vi "move_channel.vi"(4 "file index":i32=1, 6 "Mount Channel":i32=1, 8 "Desired":dbl, 9 "Device ID":refnum<vi>, 10 "Serial #":refnum<vi>, 11 "DAQ Channel":tag) -> (1 "Relative Position":waveform(dbl)[](graph) caption="Sensor Sampling", 2 "Absolute vs. Desired Position":cluster{dbl, "Position":dbl}(graph) caption="Waveform Chart", 3 "Absolute Position":dbl)   [LabVIEW 2020]
uses:
  <vilib>/Analysis/NI_AALBase.lvlib
  C:/Users/359167/Documents/LabVIEW_ws/Thorlabs.MotionControl.KCube.InertialMotorCLI.dll
  359167/Documents/LabVIEW_ws/Thorlabs.MotionControl.KCube.InertialMotorCLI.dll
  <vilib>/DAQmx/configure/timing.llb/DAQmx Timing (Sample Clock).vi
  <vilib>/DAQmx/create/channels.llb/DAQmx Create Channel (AI-Voltage-Basic).vi
  <vilib>/Utility/file.llb/Read Delimited Spreadsheet (DBL).vi
  <vilib>/Analysis/baseanly.llb/Mean (DBL).vi
  <vilib>/DAQmx/read.llb/DAQmx Read (Analog 1D Wfm NChan NSamp).vi
panel:
  out "s? t:f":string
  out "Absolute":dbl
  out "Relative (deg.)":dbl
  out "Step Size":i32
  out "Error (deg.)":dbl format="%#.3f"
  in  "Path":path=path "C:/Users/359167/Documents/saved_position.csv"
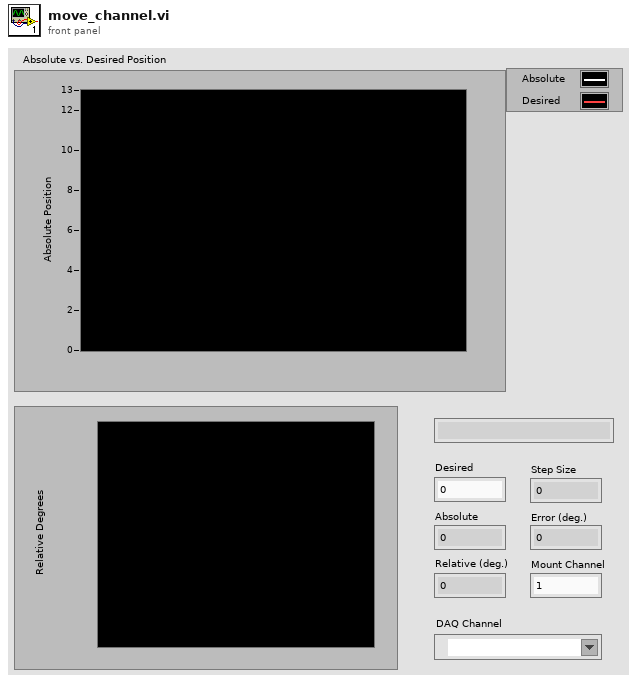
[diagram p1: front panel]
types:
  T1 = cluster{"Absolute Pos.":dbl, "Previous Deg.":dbl}
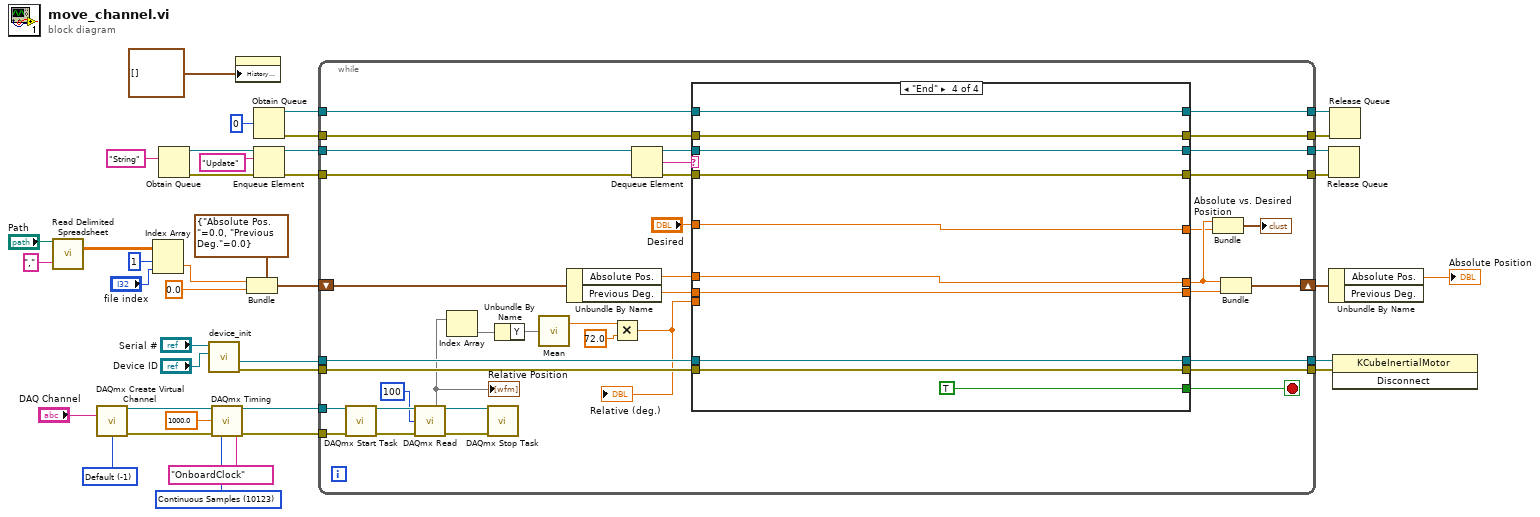
[diagram p0: block diagram]
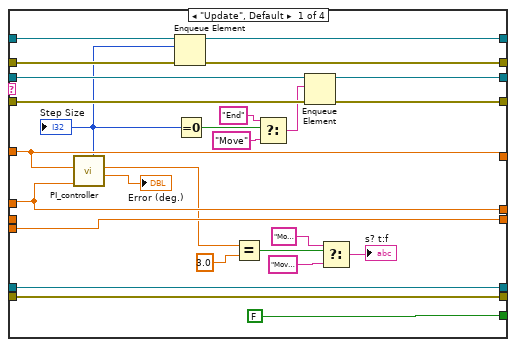
[diagram p2: hidden frame]
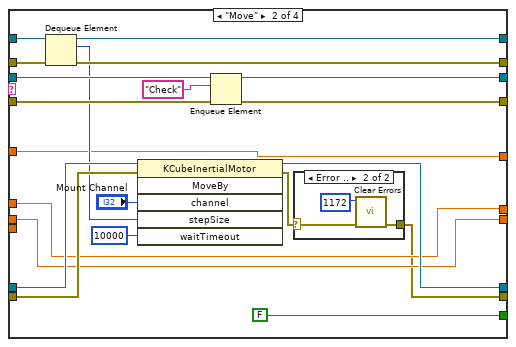
[diagram p3: hidden frame]
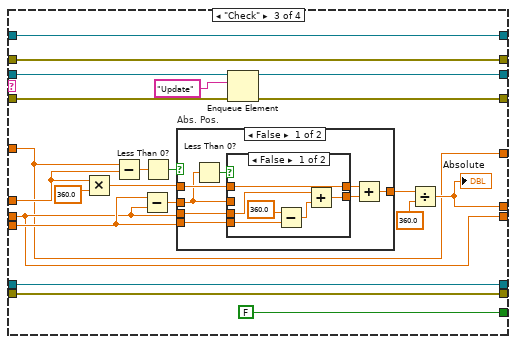
[diagram p5: hidden frame]
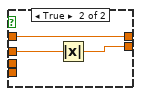
[diagram p6: hidden frame]
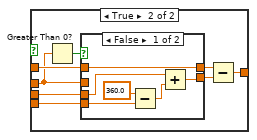
[diagram p7: hidden frame]
diagram:
  w29 = -1 items=["Default"=-1, "RSE"=10083, "NRSE"=10078, "Differential"=10106, "Pseudodifferential"=12529] ("input terminal configuration")
  w30 = 10123 items=["Finite Samples"=10178, "Continuous Samples"=10123, "Hardware Timed Single Point"=12522] ("sample mode")
  n1 = call-poly <vilib>:"Read Delimited Spreadsheet.vi"("file path (dialog if empty)"="Path", "delimiter (\\t)"="," ("delimiter (\\t)")) -> ("all rows"=w33:dbl[][])  [unwired: 8 in, 5 out]
  n2 = call-poly <vilib>:"DAQmx Create Virtual Channel.vi"("input terminal configuration"=w29, "physical channels"="DAQ Channel") -> ("task out"=w25:refnum<k21>, "error out"=w26:errorcluster)  [unwired: 12 in]
  n3 = Index Array(array=w33, index (row)=1, index (col)="file index") -> (element=w18:dbl)
  n4 = Obtain Queue(element data type="String") -> (queue out=w37:refnum<queue>, error out=w36:errorcluster)  [unwired: 4 in, 1 out]
  n5 = call "device_init.vi"("Device ID"="Device ID", "Serial #"="Serial #") -> ("error out"=w6:errorcluster, ".NET Refnum out"=w7:refnum<k24>)  [unwired: 8 in]
  n6 = call-poly <vilib>:"DAQmx Timing.vi"("task/channels in"=w25, "sample mode"=w30, "rate"=1000.0 ("sample rate"), "source"=tag "OnboardClock", "error in"=w26) -> ("task out"=w16:refnum<k21>, "error out"=w15:errorcluster)  [unwired: 9 in]
  n7 = property on="Absolute vs. Desired Position" class="WFChart (strict)"("History Data"=cluster{dbl, "Position":dbl}[] []) -> ()  [unwired: 2 in, 2 out]
  n8 = Bundle(cluster=T1 {"Absolute Pos."=0.0, "Previous Deg."=0.0}, "Absolute Pos."=w18, "Previous Deg."=0.0) -> (w17:T1)
  n9 = Obtain Queue(element data type=0) -> (queue out=w23:refnum<queue>, error out=w22:errorcluster)  [unwired: 4 in, 1 out]
  n10 = Enqueue Element(queue=w37, element="Update", error in (no error)=w36) -> (queue out=w21:refnum<queue>, error out=w20:errorcluster)  [unwired: 1 in, 1 out]
  n11 = while {
    tunnel: w23 -> [w45]
    tunnel: w22 -> [w46]
    tunnel: w20 -> [w59]
    tunnel: [w71] -> w10
    tunnel: [w62] -> w14
    tunnel: [w58] -> w13
    tunnel: [w57] -> w11
    tunnel: w21 -> [w60]
    tunnel: w16 -> [w74]
    tunnel: w15 -> [w73]
    shift-right: [w56] -> w12
    shift-left: w17 -> [w51]
    tunnel: w7 -> [w55]
    tunnel: [w72] -> w5
    tunnel: w6 -> [w54]
    tunnel: [w47] -> w4
    stop <- w76 stop-if-true
    # "Consumer"
    n12 = call <vilib>:"DAQmx Start Task.vi"("task/channels in"=w74, "error in"=w73) -> ("task out"=w67:refnum<k21>, "error out"=w68:errorcluster)  [unwired: 12 in]
    n13 = call-poly <vilib>:"DAQmx Read.vi"("task/channels in"=w67, "number of samples per channel"=100 ("n samples/channel"), "error in"=w68) -> (3:w42, "task out"=w69:refnum<k21>, "error out"=w70:errorcluster)  [unwired: 9 in, 1 out]
    "Relative Position" <- w42
    n14 = Index Array(array=w42) -> (element=w65)  [unwired: 1 in]
    n15 = call <vilib>:"DAQmx Stop Task.vi"("task/channels in"=w69, "error in"=w70) -> ()  [unwired: 12 in, 2 out]
    n16 = Unbundle By Name ("Get Waveform Components")(w65) -> ("Y"=w64)
    n17 = call-poly <vilib>:"Mean.vi"("X"=w64) -> ("mean"=w41:dbl)  [unwired: 1 out]
    n18 = Unbundle By Name(w51) -> ("Absolute Pos."=w48:dbl, "Previous Deg."=w49:dbl)
    n19 = Multiply(x=w41, y=72.0) -> (x*y=w52:dbl)
    "Relative (deg.)" <- w52
    n20 = Dequeue Element(queue=w60, error in (no error)=w59) -> (queue out=w78:refnum<queue>, element=w77:string, error out=w75:errorcluster)  [unwired: 1 in, 1 out]
    n21 = case shown="\"End\"" w77 {
      tunnel: w78 -> [w98 w124 w148 w191]
      tunnel: [w104 w119 w149 w192] -> w71
      tunnel: [FALSE FALSE FALSE TRUE] -> w76
      tunnel: w75 -> [w103 w122 w147 w192]
      tunnel: w45 -> [w102 w110 w146 w193]
      tunnel: w46 -> [w101 w109 w145 w190]
      tunnel: [w100 w108 w146 w193] -> w62
      tunnel: [w99 w107 w145 w190] -> w58
      tunnel: [w90 w125 w134 w187] -> w72
      tunnel: [w91 w112 w135 w188] -> w47
      tunnel: [w94 w121 w150 w191] -> w57
      tunnel: [w88 w114 w140 w189] -> w53
      tunnel: [w89 w113 w131 w185] -> w50
      tunnel: w55 -> [w90 w116 w134 w187]
      tunnel: w54 -> [w91 w115 w135 w188]
      tunnel: "Desired" -> [w87 w105 w130 w186]
      tunnel: w52 -> [w89 _ w133 _]
      tunnel: w48 -> [w88 w114 w132 w189]
      tunnel: w49 -> [_ w113 w131 w185]
      tunnel: [w87 w105 w130 w186] -> w43
      frame "Update", Default {
        n22 = call "PI_controller.vi"("absolute"=w88, "desired"=w87) -> ("degree error"=→"Error (deg.)":dbl, "direction"=w79:dbl, "step size"=w81:i32)  [unwired: 7 in]
        "Step Size" <- w81
        n23 = Enqueue Element(queue=w102, element=w81, error in (no error)=w101) -> (queue out=w100:refnum<queue>, error out=w99:errorcluster)  [unwired: 1 in, 1 out]
        n24 = Equal To 0?(x=w81) -> (x = 0?=w93:bool)
        n25 = Equal?(x=w79, y=3.0) -> (x = y?=w83:bool)
        n26 = Select(t="End", s=w93, f="Move" ("element")) -> (s? t:f=w95:string)
        n27 = Enqueue Element(queue=w98, element=w95, error in (no error)=w103) -> (queue out=w94:refnum<queue>, error out=w104:errorcluster)  [unwired: 1 in, 1 out]
        n28 = Select(t="Moving in reverse direction . . .", s=w83, f="Moving in forward direction . . .") -> (s? t:f=→"s? t:f":string)
      }
      frame "Move" {
        n29 = Dequeue Element(queue=w110, error in (no error)=w109) -> (queue out=w108:refnum<queue>, element=w106:i32, error out=w107:errorcluster)  [unwired: 1 in, 1 out]
        n30 = invoke class="KCubeInertialMotor" method="MoveBy"(reference=w116, error in=w115, "channel"="Mount Channel", "stepSize"=w106, "waitTimeout"=10000) -> (reference out=w125:refnum<k24>, error out=w111:errorcluster)  [unwired: 1 in, 4 out]
        n31 = Enqueue Element(queue=w124, element="Check", error in (no error)=w122) -> (queue out=w121:refnum<queue>, error out=w119:errorcluster)  [unwired: 1 in, 1 out]
        n32 = case shown="Error .." w111 {
          selector: w111 -> [w126 w128]
          tunnel: [w126 w127] -> w112
          frame No Error {
          }
          frame Error {
            n33 = call <vilib>:"Clear Errors.vi"("error in (no error)"=w128, "specific error code to clear (0: all)"=1172) -> ("error out"=w127:errorcluster)  [unwired: 4 in, 1 out]
          }
        }
      }
      frame "Check" {
        n34 = Multiply(x=w132, y=360.0) -> (x*y=w136:dbl)
        n35 = Subtract(x=w130, y=w132) -> (x-y=w139:dbl)
        n36 = Subtract(x=w133, y=w131) -> (x-y=w138:dbl)
        n37 = Less Than 0?(x=w139) -> (x < 0?=w143:bool)
        n38 = case "Abs. Pos." shown="False" w143 {
          tunnel: w136 -> [w156 w176]
          tunnel: w131 -> [w158 w174]
          tunnel: [w157 w172] -> w142
          tunnel: w133 -> [w153 w170]
          tunnel: w138 -> [w152 w169]
          frame False {
            n39 = Less Than 0?(x=w152) -> (x < 0?=w159:bool)
            n40 = case shown="False" w159 {
              tunnel: w156 -> [w165 w168]
              tunnel: [w160 w166] -> w154
              tunnel: w158 -> [w161 _]
              tunnel: w153 -> [w163 _]
              tunnel: [w165 w168] -> w155
              tunnel: w152 -> [_ w167]
              frame False {
                n41 = Subtract(x=360.0 ("y"), y=w163) -> (x-y=w162:dbl)
                n42 = Add(x=w161, y=w162) -> (x+y=w160:dbl)
              }
              frame True {
                n43 = Absolute Value(x=w167) -> (abs(x)=w166:dbl)
              }
            }
            n44 = Add(x=w155, y=w154) -> (x+y=w157:dbl)
          }
          frame True {
            n45 = Greater Than 0?(x=w169) -> (x > 0?=w175:bool)
            n46 = case shown="False" w175 {
              tunnel: w176 -> [w179 w184]
              tunnel: w169 -> [_ w183]
              tunnel: w174 -> [w182 _]
              tunnel: [w180 w183] -> w173
              tunnel: [w179 w184] -> w171
              tunnel: w170 -> [w177 _]
              frame False {
                n47 = Subtract(x=360.0, y=w177) -> (x-y=w181:dbl)
                n48 = Add(x=w182, y=w181) -> (x+y=w180:dbl)
              }
              frame True {
              }
            }
            n49 = Subtract(x=w171, y=w173) -> (x-y=w172:dbl)
          }
        }
        n50 = Enqueue Element(queue=w148, element="Update", error in (no error)=w147) -> (queue out=w150:refnum<queue>, error out=w149:errorcluster)  [unwired: 1 in, 1 out]
        n51 = Divide ("absolute position")(x=w142, y=360.0) -> (x/y=w140:dbl)
        "Absolute" <- w140
      }
      frame "End" {
      }
    }
    n52 = Bundle("Absolute Pos."=w53, "Desired"=w43) -> (→"Absolute vs. Desired Position":cluster{"Absolute Pos.":dbl, "Desired":dbl})  [unwired: 1 in]
    n53 = Bundle("Absolute Pos."=w53, "Previous Deg."=w50) -> (w56:T1)  [unwired: 1 in]
  }
  n54 = Release Queue(queue=w11, error in (no error)=w10) -> ()  [unwired: 1 in, 3 out]
  n55 = Unbundle By Name(w12) -> ("Absolute Pos."=→"Absolute Position":dbl)  [unwired: 1 out]
  n56 = Release Queue(queue=w14, error in (no error)=w13) -> ()  [unwired: 1 in, 3 out]
  n57 = invoke class="KCubeInertialMotor" method="Disconnect"(reference=w5, error in=w4) -> ()  [unwired: 1 in, 3 out]
